vi "AIM664 UDP Block Write.vi"() -> ()   [LabVIEW 2020]
uses:
  src/AIM664LV.lvlib
panel:
  out "error out":errorcluster
  out "ResourceInfo 2":T1 {"PortMode" items=[" FDX_SINGLE", "FDX_REDUNDANT"]}
  out "ResourceInfo":T1 {"PortMode" items=[" FDX_SINGLE", "FDX_REDUNDANT"]}
  out "output cluster":T2={"GlobalResultCode"=0, "MsgCountOut"=2, "UdpBlockWriteResultArray"=[942640, 33, 0, 951280, 37, 0, 0, 0, 0, 0, 0, 0, 0, 0, 0, 0, 0, 0, 0, 0, 0, 0, 0, 0, 0, 0, 0, 0, 0, 0, 0, 0, 0, 0, 0, 0, 0, 0, 0, 0, 0, 0, 0, 0, 0, 0, 0, 0, 0, 0, 0, 0, 0, 0, 0, 0, 0, 0, 0, 0, 0, 0, 0, 0, 0, 0, 0, 0, 0, 0, 0, 0, 0, 0, 0, 0, 0, 0, 0, 0, 0, 0, 0, 0, 0, 0, 0, 0, 0, 0, 0, 0, 0, 0, 0, 0, 0, 0, 0, 0]}
  in  "Array 2":u32[](array[numeric])=[286331153, 572662306, 858993459, 1145324612, 1431655765, 1717986918, 2004318071, 2290649224, 2576980377, 170] format="%x"
  in  "Array":u32[](array[numeric])=[1985229328, 4275878552, 1985229328, 4275878552, 1985229328, 4275878552, 1985229328, 4275878552, 16] format="%x"
  in  "UDP Create Port2":T3={"PortType"=0, "UdpSrc"=2, "IpSrc"=167846145, "VlId"=0, "IpDst"=3772776448, "UdpDst"=2, "UdpNumBufMessages"=1, "UdpSamplingRate"=8, "UdpMaxMessageSize"=40, "SubVlId"=2} {"IpDst" format="%x"; "IpSrc" format="%x"}
  in  "UDP Create Port1":T3={"PortType"=0, "UdpSrc"=1, "IpSrc"=167846145, "VlId"=0, "IpDst"=3772776448, "UdpDst"=1, "UdpNumBufMessages"=1, "UdpSamplingRate"=8, "UdpMaxMessageSize"=40, "SubVlId"=1} {"IpDst" format="%x"; "IpSrc" format="%x"}
  in  "VL Control":T4={"MaxFrameLength"=300, "FrameBufferSize"=300, "MACSourceLSLW"=563904, "VlId"=0, "SubVls"=2, "Bag"=16, "NetSelect"=3, "MACSourceMSLW"=512, "Skew"=0} {"MACSourceMSLW" format="%x"; "NetSelect" items=["FDX_TX_FRAME_DLY_A"=0, "FDX_TX_FRAME_DLY_B"=1, "FDX_TX_FRAME_BOTH "=3, "FDX_TX_FRAME_ONLY_A"=4, "FDX_TX_FRAME_ONLY_B "=5]; "MACSourceLSLW" format="%x"}
  in  "Input Cluster 2":T5 {"ExtendedStopMode" items=["FDX_ESTOP_NOT_USED", "FDX_ESTOP_EXT_TRG", "FDX_ESTOP_EXT_TRG_RESTART", "FDX_ESTOP_TIME"]; "StartMode" items=["FDX_STOP", "FDX_START", "FDX_START_TRG", "FDX_START_TIME"]}
  in  "Input Cluster":T5={"StartMode"=1, "Count"=100, "Sign"=0, "Day"=0, "Hour"=0, "Min"=0, "Second"=0, "MilliSec"=0, "MicroSec"=0, "ExtendedStopMode"=0, "TransmitTime"=0} {"ExtendedStopMode" items=["FDX_ESTOP_NOT_USED", "FDX_ESTOP_EXT_TRG", "FDX_ESTOP_EXT_TRG_RESTART", "FDX_ESTOP_TIME"]; "StartMode" items=["FDX_STOP", "FDX_START", "FDX_START_TRG", "FDX_START_TIME"]}
  in  "Input Cluster":T6={"SrvName"="local", "ClHostName"="local", "ClUser"="Brett", "ClApplication"="Test", "ClApplicationVersion"="V01.00", "ResourceID"=1, "Privileges"=4294967295} {"Privileges" items=["PRIVILEGES_ADMIN"=4294967295]}
  in  "Input Cluster":T7={"SrvName"="local", "ResourceID"=1, "ResourceType"=0} {"ResourceType" items=["Board", "Port"]}
  out "Output Cluster 2":T8={"ResourceID"=1, "ResourceType"=0, "ResourceInfo"="AMC-FDX-B2", "StructId"=0}
  in  "ServerRElement":u32=1
  in  "PortMap":u32=1
  out "Output Cluster":T9={"PortConfig"=0, "PortUsed"=1, "GlobalMemFree"=62889696, "SharedMemFree"=16566232} {"PortConfig" items=["FDX_SINGLE", "FDX_REDUNDANT"]}
  out "Output Cluster":T10={"Frames"=97, "TxStatus"=1, "TransmitMode"=2, "FramesPortB"=0} {"TransmitMode" items=["FDX_TX_GENERIC", "FDX_TX_REPLAY", "FDX_TX_INDIVIDUAL"]; "TxStatus" items=["FDX_STAT_STOP", "FDX_STAT_RUN", "FDX_STAT_ERROR", "FDX_STAT_WAIT_F_TRIG"]}
  in  "RerosPortDelay":u32
  in  "TransmitMode":u32(ring)=2 items=["FDX_TX_GENERIC", "FDX_TX_REPLAY", "FDX_TX_INDIVIDUAL"]
  in  "Input Cluster":T7={"SrvName"="local", "ResourceID"=2, "ResourceType"=1} {"ResourceType" items=["Board", "Port"]}
  in  "Input Cluster":T6={"SrvName"="local", "ClHostName"="local", "ClUser"="Brett", "ClApplication"="Test", "ClApplicationVersion"="V01.00", "ResourceID"=2, "Privileges"=4294967295} {"Privileges" items=["PRIVILEGES_ADMIN"=4294967295]}
  out "Output Cluster":T8={"ResourceID"=1, "ResourceType"=0, "ResourceInfo"="AMC-FDX-B2", "StructId"=0}
  in  "ServerRElement":u32=1
  out "NuOfResources":u32=3
  in  "SrvName":string="local"
  out "NuOfServers":u32=1
  # "ARINC 664 UDP Block Write"
  # "Overview: Configure the board to write UDP blocks into a Port.\nRequirement: At least one AIM ARINC-664 board with installed AIM ARINC 664 BSP.\nRestrictions: None.\nInstruction:\n1. Run the VI.\n2. Verify the results in the indicators."
  # "Tx Port"
  # "Board"
  # "Board"
  # "Tx Port"
  # "FdxTxPortInitCvi"
  # "FdxTxModeControlCvi"
  # "FdxTxCreateVLCvi"
  # "FdxTxUDPCreatePortCvi"
  # "FdxTxUDPCreatePortCvi"
  # "FdxLogoutCvi"
  # "FdxLogoutCvi"
  # "FdxTxControlCvi"
  # "FdxTxStatusCvi"
  # "FdxTxControlCvi"
  # "FdxTxUDPBlockWriteCvi"
  # "FdxInitCvi"
  # "CountServerResourcesCvi"
  # "GetServerResourcesCvi"
  # "QueryServerResourceCvi"
  # "FdxLoginCvi"
  # "GetServerResourcesCvi"
  # "QueryServerResourceCvi"
  # "FdxLoginCvi"
  # "Input"
  # "Input"
  # "Input"
  # "Input"
  # "Input"
  # "Input"
  # "Input"
  # "Input"
  # "Input"
  # "Input"
  # "Input"
  # "Input"
  # "Output"
  # "Input"
  # "Output"
  # "Output"
  # "Output"
  # "Output"
  # "Output"
  # "Output"
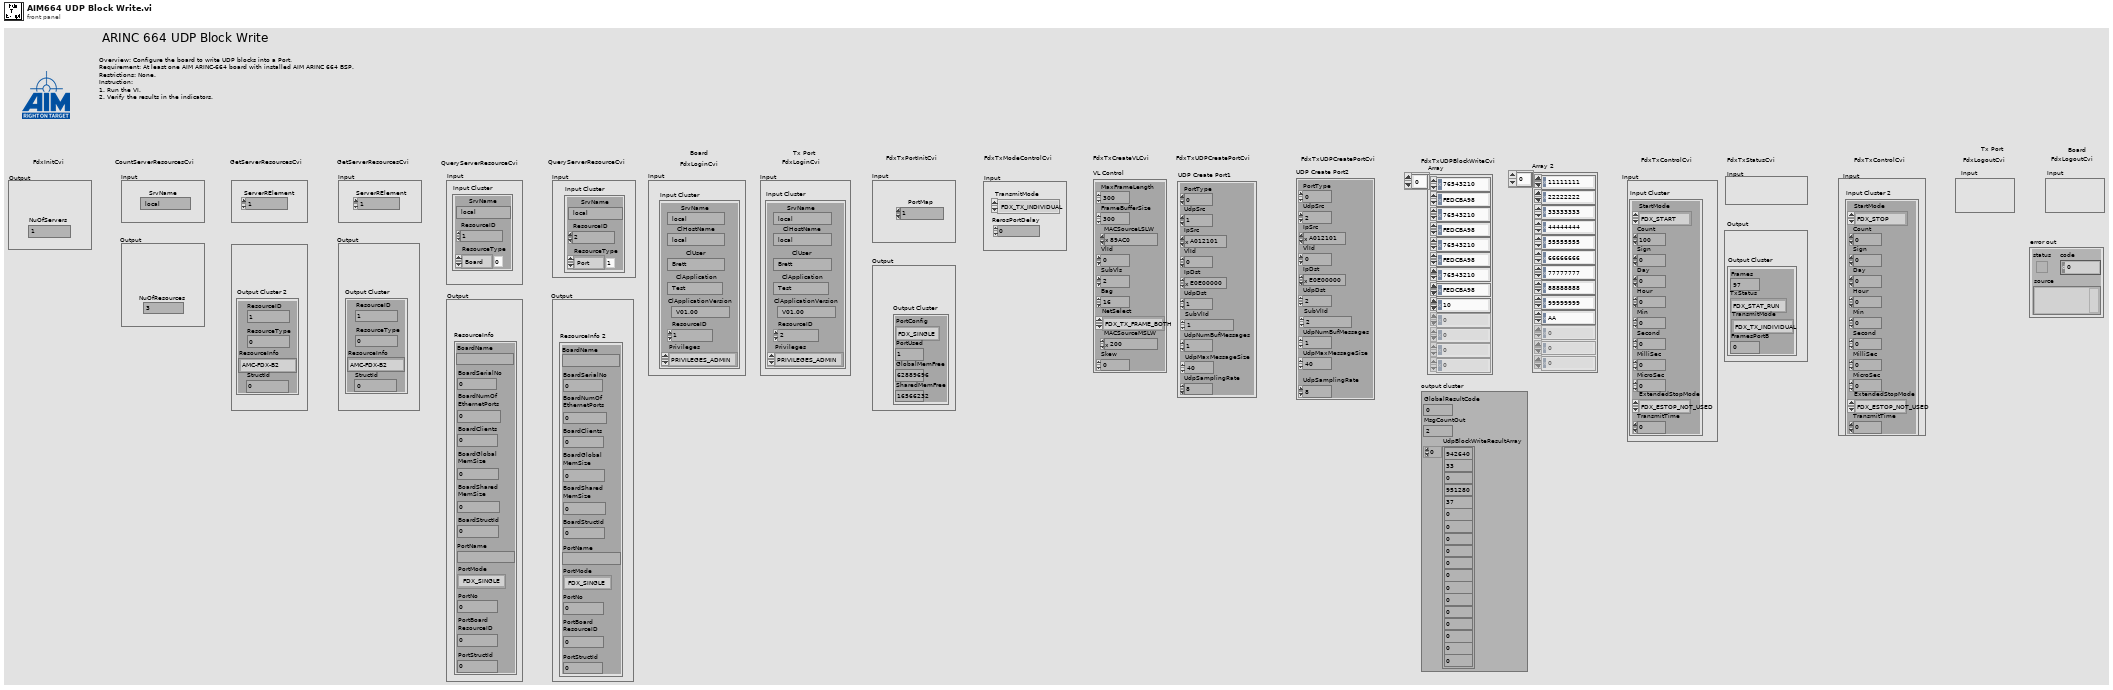
[diagram p1: front panel]
types:
  T1 = cluster{"BoardName":string, "BoardSerialNo":u32, "BoardNumOf\nEthernetPorts":u32, "BoardClients":u32, "BoardGlobal\nMemSize":u32, "BoardShared\nMemSize":u32, "BoardStructId":u32, "PortName":string, "PortMode":u32, "PortNo":u32, "PortBoard\nResourceID":u32, "PortStructId":u32}
  T2 = cluster{"GlobalResultCode":i32, "MsgCountOut":u32, "UdpBlockWriteResultArray":u32[]}
  T3 = cluster{"PortType":u32, "UdpSrc":u32, "IpSrc":u32, "VlId":u32, "IpDst":u32, "UdpDst":u32, "UdpNumBufMessages":u32, "UdpSamplingRate":u32, "UdpMaxMessageSize":u32, "SubVlId":u32}
  T4 = cluster{"MaxFrameLength":u32, "FrameBufferSize":u32, "MACSourceLSLW":u32, "VlId":u32, "SubVls":u32, "Bag":u32, "NetSelect":u32, "MACSourceMSLW":u32, "Skew":u32}
  T5 = cluster{"StartMode":i32, "Count":u32, "Sign":i32, "Day":u32, "Hour":u32, "Min":u32, "Second":u32, "MilliSec":u32, "MicroSec":u32, "ExtendedStopMode":i32, "TransmitTime":u32}
  T6 = cluster{"SrvName":string, "ClHostName":string, "ClUser":string, "ClApplication":string, "ClApplicationVersion":string, "ResourceID":u32, "Privileges":u32}
  T7 = cluster{"SrvName":string, "ResourceID":u32, "ResourceType":u32}
  T8 = cluster{"ResourceID":u32, "ResourceType":u32, "ResourceInfo":string, "StructId":u32}
  T9 = cluster{"PortConfig":u32, "PortUsed":u32, "GlobalMemFree":u32, "SharedMemFree":u32}
  T10 = cluster{"Frames":u32, "TxStatus":i32, "TransmitMode":u32, "FramesPortB":u32}
  T11 = cluster{"TxStatus":u32, "Frames":u32, "TransmitMode":u32, "FramesPortB":u32}
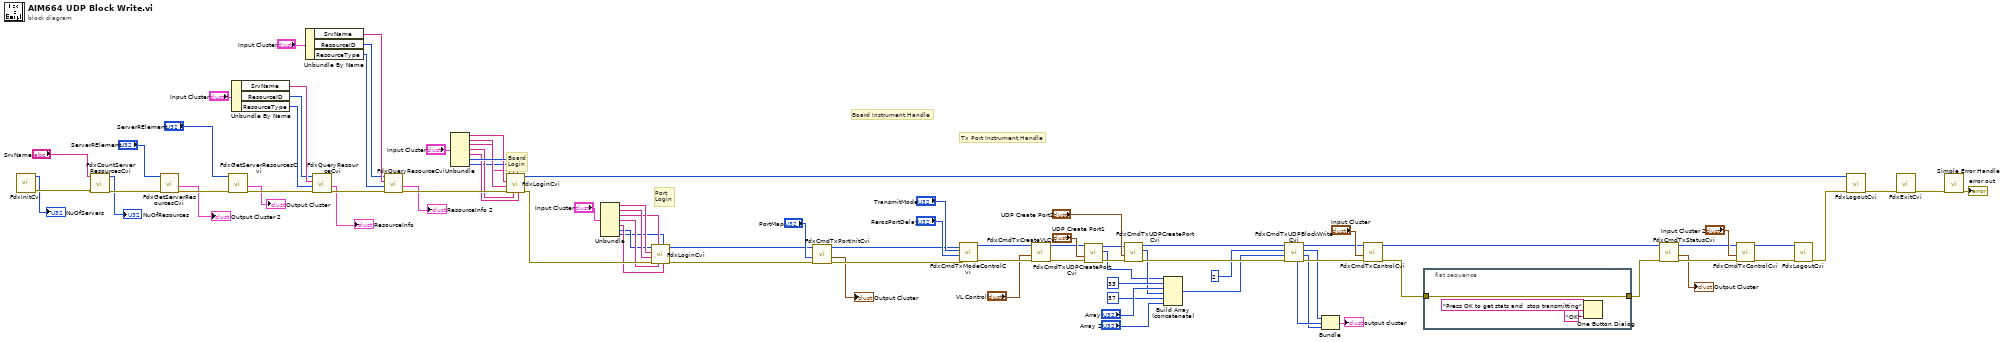
[diagram p0: block diagram]
diagram:
  # "Tx Port Instrument Handle"
  # "Board Instrument Handle"
  # "Port\nLogin"
  # "Board\nLogin"
  n1 = call "FdxInitCvi.vi"() -> ("error out"=w84:errorcluster, "Number of Servers"=→"NuOfServers":u32)  [unwired: 10 in]
  n2 = call "FdxCountServerResourcesCvi.vi"("error in"=w84, "SrvName (local)"="SrvName") -> ("error out"=w83:errorcluster, "Number of Resources"=→"NuOfResources":u32)  [unwired: 8 in]
  n3 = call "FdxGetServerResourcesCvi.vi"("error in"=w83, "ServerRElement"="ServerRElement") -> ("error out"=w82:errorcluster, "ServerResourceInfo"=→"Output Cluster 2":T8)  [unwired: 4 in, 4 out]
  n4 = call "FdxGetServerResourcesCvi.vi"("error in"=w82, "ServerRElement"="ServerRElement") -> ("error out"=w88:errorcluster, "ServerResourceInfo"=→"Output Cluster":T8)  [unwired: 4 in, 4 out]
  n5 = Unbundle By Name("Input Cluster") -> ("SrvName"=w36:string, "ResourceID"=w35:u32, "ResourceType"=w34:u32)
  n6 = Unbundle By Name("Input Cluster") -> ("SrvName"=w32:string, "ResourceID"=w31:u32, "ResourceType"=w30:u32)
  n7 = call "FdxQueryResourceCvi.vi"("error in"=w88, "ResourceType"=w34, "SrvName"=w36, "ResourceID"=w35) -> ("error out"=w81:errorcluster, "ResourceInfo"=→"ResourceInfo":T1)  [unwired: 5 in, 1 out]
  n8 = call "FdxQueryResourceCvi.vi"("error in"=w81, "ResourceType"=w30, "SrvName"=w32, "ResourceID"=w31) -> ("error out"=w80:errorcluster, "ResourceInfo"=→"ResourceInfo 2":T1)  [unwired: 5 in, 1 out]
  n9 = Unbundle("Input Cluster") -> ("SrvName"=w19:string, "ClHostName"=w18:string, "ClUser"=w17:string, "ClApplication"=w16:string, "ClApplicationVersion"=w15:string, "ResourceID"=w20:u32, "Privileges"=w14:u32)
  n10 = call "FdxLoginCvi.vi"("ClApplicationVersion"=w15, "Privileges"=w14, "ClApplication"=w16, "ClUser"=w17, "error in"=w80, "ClHostName"=w18, "SrvName"=w19, "ResourceID"=w20) -> ("error out"=w79:errorcluster, "InstrumentHandle"=w48:u32)  [unwired: 2 in]
  n11 = Unbundle("Input Cluster") -> ("SrvName"=w28:string, "ClHostName"=w27:string, "ClUser"=w26:string, "ClApplication"=w25:string, "ClApplicationVersion"=w24:string, "ResourceID"=w23:u32, "Privileges"=w22:u32)
  n12 = call "FdxLoginCvi.vi"("ClApplicationVersion"=w24, "Privileges"=w22, "ClApplication"=w25, "ClUser"=w26, "error in"=w79, "ClHostName"=w27, "SrvName"=w28, "ResourceID"=w23) -> ("error out"=w70:errorcluster, "InstrumentHandle"=w41:u32)  [unwired: 2 in]
  n13 = call "FdxCmdTxPortInitCvi.vi"("error in"=w70, "PortMap"="PortMap", "InstrumentHandle_port"=w41) -> ("error out"=w87:errorcluster, "PortInitOut"=→"Output Cluster":T9, "InstrumentHandle_port"=w47:u32)  [unwired: 6 in]
  n14 = call "FdxCmdTxModeControlCvi.vi"("error in"=w87, "RerosPortDelay"="RerosPortDelay", "TransmitMode"="TransmitMode", "InstrumentHandle_port"=w47) -> ("error out"=w75:errorcluster, "InstrumentHandle_port"=w46:u32)  [unwired: 6 in]
  n15 = call "FdxCmdTxCreateVLCvi.vi"("error in"=w75, "Input Cluster"="VL Control", "InstrumentHandle_port"=w46) -> ("error out"=w74:errorcluster, "InstrumentHandle_port"=w45:u32)  [unwired: 7 in]
  n16 = call "FdxCmdTxUDPCreatePortCvi.vi"("error in"=w74, "UdpDescription"="UDP Create Port1", "InstrumentHandle"=w45) -> ("error out"=w73:errorcluster, "UdpHandle"=w3:u32, "InstrumentHandle"=w44:u32)  [unwired: 6 in]
  n17 = call "FdxCmdTxUDPCreatePortCvi.vi"("error in"=w73, "UdpDescription"="UDP Create Port2", "InstrumentHandle"=w44) -> ("error out"=w71:errorcluster, "UdpHandle"=w10:u32, "InstrumentHandle"=w43:u32)  [unwired: 6 in]
  n18 = Build Array (concatenate)(w3, u32 33 ("element"), "Array", w10, u32 37 ("element"), "Array 2") -> (w4:u32[])
  n19 = call "FdxCmdTxUDPBlockWriteCvi.vi"("error in"=w71, "UdpBlockWriteMsgArray"=w4, "MsgCount"=u32 2, "InstrumentHandle"=w43) -> ("error out"=w72:errorcluster, "UdpBlockWriteResultArray"=w6:u32[], "GlobalResultCode"=w8:i32, "InstrumentHandle"=w42:u32, "MsgCountOut"=w7:u32)  [unwired: 3 in]
  n20 = Bundle("GlobalResultCode"=w8, "MsgCountOut"=w7, "UdpBlockWriteResultArray"=w6) -> (→"output cluster":T2)  [unwired: 1 in]
  n21 = call "FdxCmdTxControlCvi.vi"("error in"=w72, "TxControl"="Input Cluster", "InstrumentHandle_port"=w42) -> ("error out"=w86:errorcluster, "InstrumentHandle_port"=w40:u32)  [unwired: 7 in]
  n22 = flat-sequence {
    tunnel: w86 -> [w91]
    tunnel: [w91] -> w85
    frame #0 {
      n23 = One Button Dialog(message="Press OK to get stats and  stop transmitting", button name ("OK")="OK") -> ()  [unwired: 1 out]
    }
  }
  n24 = call "FdxCmdTxStatusCvi.vi"("error in"=w85, "InstrumentHandle_port"=w40) -> ("error out"=w78:errorcluster, "TxStatus"=→"Output Cluster":T11, "InstrumentHandle_port"=w39:u32)  [unwired: 7 in]
  n25 = call "FdxCmdTxControlCvi.vi"("error in"=w78, "TxControl"="Input Cluster 2", "InstrumentHandle_port"=w39) -> ("error out"=w76:errorcluster, "InstrumentHandle_port"=w38:u32)  [unwired: 7 in]
  n26 = call "FdxLogoutCvi.vi"("error in"=w76, "InstrumentHandle"=w38) -> ("error out"=w77:errorcluster)  [unwired: 9 in]
  n27 = call "FdxLogoutCvi.vi"("error in"=w77, "InstrumentHandle"=w48) -> ("error out"=w69:errorcluster)  [unwired: 9 in]
  n28 = call "FdxExitCvi.vi"("error in"=w69) -> ("error out"=w2:errorcluster)  [unwired: 10 in]
  n29 = call <vilib>:"Simple Error Handler.vi"("error in (no error)"=w2) -> ("error out"=→"error out":errorcluster)  [unwired: 4 in, 4 out]
